vi "Profile_Write.vi"(8 "error in":errorcluster, 10 "Configuration Cluster":T1={"General"={"Config.ini"=path "", "Default Logging Path"=path ""}, "Hardware"={"LCR VISA COM"="", "Measure Rate (1/s)"=0, "Reset on Load?"=FALSE, "Measure Profile"=path "", "Global T VAR"="", "Global B VAR"=""}, "HM8118 Current Profile"={"Bias Profile"={" Bias Source (OFF)"=0, " Bias Type (Voltage)"=0, "Bias Level (0)"=0.0}, "Measurement Profile"={"Operation Mode (0: Auto)"=0, "Circuit Type (2: Auto)"=2, "Manual Range (1:Range 1 and 25 Ohms)"=1, "Auto Range (T: Enable)"=TRUE}, "Signal Profile"={"Frequency (1kHz)"=1000.0, "Measuring Voltage (1V)"=1.0}, "Integration Profile"={"Averaging (0: Off)"=0, "Averaging Number (2)"=2, "Time (100ms)"=100, "Rate (0: Fast)"=0}, "Trigger Profile"={"Trigger Mode (0: Continuous)"=0}}, "HM8118 New Profile"={"Bias Profile"={" Bias Source (OFF)"=0, " Bias Type (Voltage)"=0, "Bias Level (0)"=0.0}, "Measurement Profile"={"Operation Mode (0: Auto)"=0, "Circuit Type (2: Auto)"=2, "Manual Range (1:Range 1 and 25 Ohms)"=1, "Auto Range (T: Enable)"=TRUE}, "Signal Profile"={"Frequency (1kHz)"=1000.0, "Measuring Voltage (1V)"=1.0}, "Integration Profile"={"Averaging (0: Off)"=0, "Averaging Number (2)"=2, "Time (100ms)"=100, "Rate (0: Fast)"=0}, "Trigger Profile"={"Trigger Mode (0: Continuous)"=0}}, "Operation"={"Operation Mode"=enum."Idle-Off", "Status"="", "NewLog?"=FALSE}} {"HM8118 New Profile"."Trigger Profile"."Trigger Mode (0: Continuous)" items=["Continuous", "Manual", "External"]; "HM8118 New Profile"."Integration Profile"."Rate (0: Fast)" items=["Fast", "Medium", "Slow"]; "HM8118 New Profile"."Integration Profile"."Time (100ms)" min=1 max=999; "HM8118 New Profile"."Integration Profile"."Averaging Number (2)" min=2 max=99; "HM8118 New Profile"."Integration Profile"."Averaging (0: Off)" items=["Off", "Normal", "Averaging"]; "HM8118 New Profile"."Signal Profile"."Measuring Voltage (1V)" min=0.05 max=1.5 step=0.01; "HM8118 New Profile"."Signal Profile"."Frequency (1kHz)" min=20.0 max=200000.0; "HM8118 New Profile"."Measurement Profile"."Manual Range (1:Range 1 and 25 Ohms)" items=["Range 1 and 25 Ohms"=1, "Range 2 and 25 Ohms"=2, "Range 3 and 400 Ohms"=3, "Range 4 and 6.4 kOhms"=4, "Range 5 and 100kOhms"=5, "Range 6 and 100kOhms"=6]; "HM8118 New Profile"."Measurement Profile"."Circuit Type (2: Auto)" items=["Series", "Parallel", "Auto"]; "HM8118 New Profile"."Measurement Profile"."Operation Mode (0: Auto)" items=["Auto", "L+Q", "L+R", "C+D", "C+R", "R+Q", "Z+Theta", "Y+Theta", "R+X", "G+B", "N+Theta", "M"]; "HM8118 New Profile"."Bias Profile"."Bias Type (Voltage)" items=["Voltage", "Current"]; "HM8118 New Profile"."Bias Profile"."Bias Source (OFF)" items=["Off", "Internal", "External"]; "HM8118 Current Profile"."Trigger Profile"."Trigger Mode (0: Continuous)" items=["Continuous", "Manual", "External"]; "HM8118 Current Profile"."Integration Profile"."Rate (0: Fast)" items=["Fast", "Medium", "Slow"]; "HM8118 Current Profile"."Integration Profile"."Time (100ms)" min=1 max=999; "HM8118 Current Profile"."Integration Profile"."Averaging Number (2)" min=2 max=99; "HM8118 Current Profile"."Integration Profile"."Averaging (0: Off)" items=["Off", "Normal", "Averaging"]; "HM8118 Current Profile"."Signal Profile"."Measuring Voltage (1V)" min=0.05 max=1.5 step=0.01; "HM8118 Current Profile"."Signal Profile"."Frequency (1kHz)" min=20.0 max=200000.0; "HM8118 Current Profile"."Measurement Profile"."Manual Range (1:Range 1 and 25 Ohms)" items=["Range 1 and 25 Ohms"=1, "Range 2 and 25 Ohms"=2, "Range 3 and 400 Ohms"=3, "Range 4 and 6.4 kOhms"=4, "Range 5 and 100kOhms"=5, "Range 6 and 100kOhms"=6]; "HM8118 Current Profile"."Measurement Profile"."Circuit Type (2: Auto)" items=["Series", "Parallel", "Auto"]; "HM8118 Current Profile"."Measurement Profile"."Operation Mode (0: Auto)" items=["Auto", "L+Q", "L+R", "C+D", "C+R", "R+Q", "Z+Theta", "Y+Theta", "R+X", "G+B", "N+Theta", "M"]; "HM8118 Current Profile"."Bias Profile"."Bias Type (Voltage)" items=["Voltage", "Current"]; "HM8118 Current Profile"."Bias Profile"."Bias Source (OFF)" items=["Off", "Internal", "External"]}) -> (0 "error out":errorcluster, 2 "Configuration Cluster Out":T1={"General"={"Config.ini"=path "", "Default Logging Path"=path ""}, "Hardware"={"LCR VISA COM"="", "Measure Rate (1/s)"=0, "Reset on Load?"=FALSE, "Measure Profile"=path "", "Global T VAR"="", "Global B VAR"=""}, "HM8118 Current Profile"={"Bias Profile"={" Bias Source (OFF)"=0, " Bias Type (Voltage)"=0, "Bias Level (0)"=0.0}, "Measurement Profile"={"Operation Mode (0: Auto)"=0, "Circuit Type (2: Auto)"=2, "Manual Range (1:Range 1 and 25 Ohms)"=1, "Auto Range (T: Enable)"=TRUE}, "Signal Profile"={"Frequency (1kHz)"=1000.0, "Measuring Voltage (1V)"=1.0}, "Integration Profile"={"Averaging (0: Off)"=0, "Averaging Number (2)"=2, "Time (100ms)"=100, "Rate (0: Fast)"=0}, "Trigger Profile"={"Trigger Mode (0: Continuous)"=0}}, "HM8118 New Profile"={"Bias Profile"={" Bias Source (OFF)"=0, " Bias Type (Voltage)"=0, "Bias Level (0)"=0.0}, "Measurement Profile"={"Operation Mode (0: Auto)"=0, "Circuit Type (2: Auto)"=2, "Manual Range (1:Range 1 and 25 Ohms)"=1, "Auto Range (T: Enable)"=TRUE}, "Signal Profile"={"Frequency (1kHz)"=1000.0, "Measuring Voltage (1V)"=1.0}, "Integration Profile"={"Averaging (0: Off)"=0, "Averaging Number (2)"=2, "Time (100ms)"=100, "Rate (0: Fast)"=0}, "Trigger Profile"={"Trigger Mode (0: Continuous)"=0}}, "Operation"={"Operation Mode"=enum."Idle-Off", "Status"="", "NewLog?"=FALSE}} {"HM8118 New Profile"."Trigger Profile"."Trigger Mode (0: Continuous)" items=["Continuous", "Manual", "External"]; "HM8118 New Profile"."Integration Profile"."Rate (0: Fast)" items=["Fast", "Medium", "Slow"]; "HM8118 New Profile"."Integration Profile"."Time (100ms)" min=1 max=999; "HM8118 New Profile"."Integration Profile"."Averaging Number (2)" min=2 max=99; "HM8118 New Profile"."Integration Profile"."Averaging (0: Off)" items=["Off", "Normal", "Averaging"]; "HM8118 New Profile"."Signal Profile"."Measuring Voltage (1V)" min=0.05 max=1.5 step=0.01; "HM8118 New Profile"."Signal Profile"."Frequency (1kHz)" min=20.0 max=200000.0; "HM8118 New Profile"."Measurement Profile"."Manual Range (1:Range 1 and 25 Ohms)" items=["Range 1 and 25 Ohms"=1, "Range 2 and 25 Ohms"=2, "Range 3 and 400 Ohms"=3, "Range 4 and 6.4 kOhms"=4, "Range 5 and 100kOhms"=5, "Range 6 and 100kOhms"=6]; "HM8118 New Profile"."Measurement Profile"."Circuit Type (2: Auto)" items=["Series", "Parallel", "Auto"]; "HM8118 New Profile"."Measurement Profile"."Operation Mode (0: Auto)" items=["Auto", "L+Q", "L+R", "C+D", "C+R", "R+Q", "Z+Theta", "Y+Theta", "R+X", "G+B", "N+Theta", "M"]; "HM8118 New Profile"."Bias Profile"."Bias Type (Voltage)" items=["Voltage", "Current"]; "HM8118 New Profile"."Bias Profile"."Bias Source (OFF)" items=["Off", "Internal", "External"]; "HM8118 Current Profile"."Trigger Profile"."Trigger Mode (0: Continuous)" items=["Continuous", "Manual", "External"]; "HM8118 Current Profile"."Integration Profile"."Rate (0: Fast)" items=["Fast", "Medium", "Slow"]; "HM8118 Current Profile"."Integration Profile"."Time (100ms)" min=1 max=999; "HM8118 Current Profile"."Integration Profile"."Averaging Number (2)" min=2 max=99; "HM8118 Current Profile"."Integration Profile"."Averaging (0: Off)" items=["Off", "Normal", "Averaging"]; "HM8118 Current Profile"."Signal Profile"."Measuring Voltage (1V)" min=0.05 max=1.5 step=0.01; "HM8118 Current Profile"."Signal Profile"."Frequency (1kHz)" min=20.0 max=200000.0; "HM8118 Current Profile"."Measurement Profile"."Manual Range (1:Range 1 and 25 Ohms)" items=["Range 1 and 25 Ohms"=1, "Range 2 and 25 Ohms"=2, "Range 3 and 400 Ohms"=3, "Range 4 and 6.4 kOhms"=4, "Range 5 and 100kOhms"=5, "Range 6 and 100kOhms"=6]; "HM8118 Current Profile"."Measurement Profile"."Circuit Type (2: Auto)" items=["Series", "Parallel", "Auto"]; "HM8118 Current Profile"."Measurement Profile"."Operation Mode (0: Auto)" items=["Auto", "L+Q", "L+R", "C+D", "C+R", "R+Q", "Z+Theta", "Y+Theta", "R+X", "G+B", "N+Theta", "M"]; "HM8118 Current Profile"."Bias Profile"."Bias Type (Voltage)" items=["Voltage", "Current"]; "HM8118 Current Profile"."Bias Profile"."Bias Source (OFF)" items=["Off", "Internal", "External"]})   [LabVIEW 2021]
uses:
  Config_Cluster.ctl
  Mode_Enum.ctl
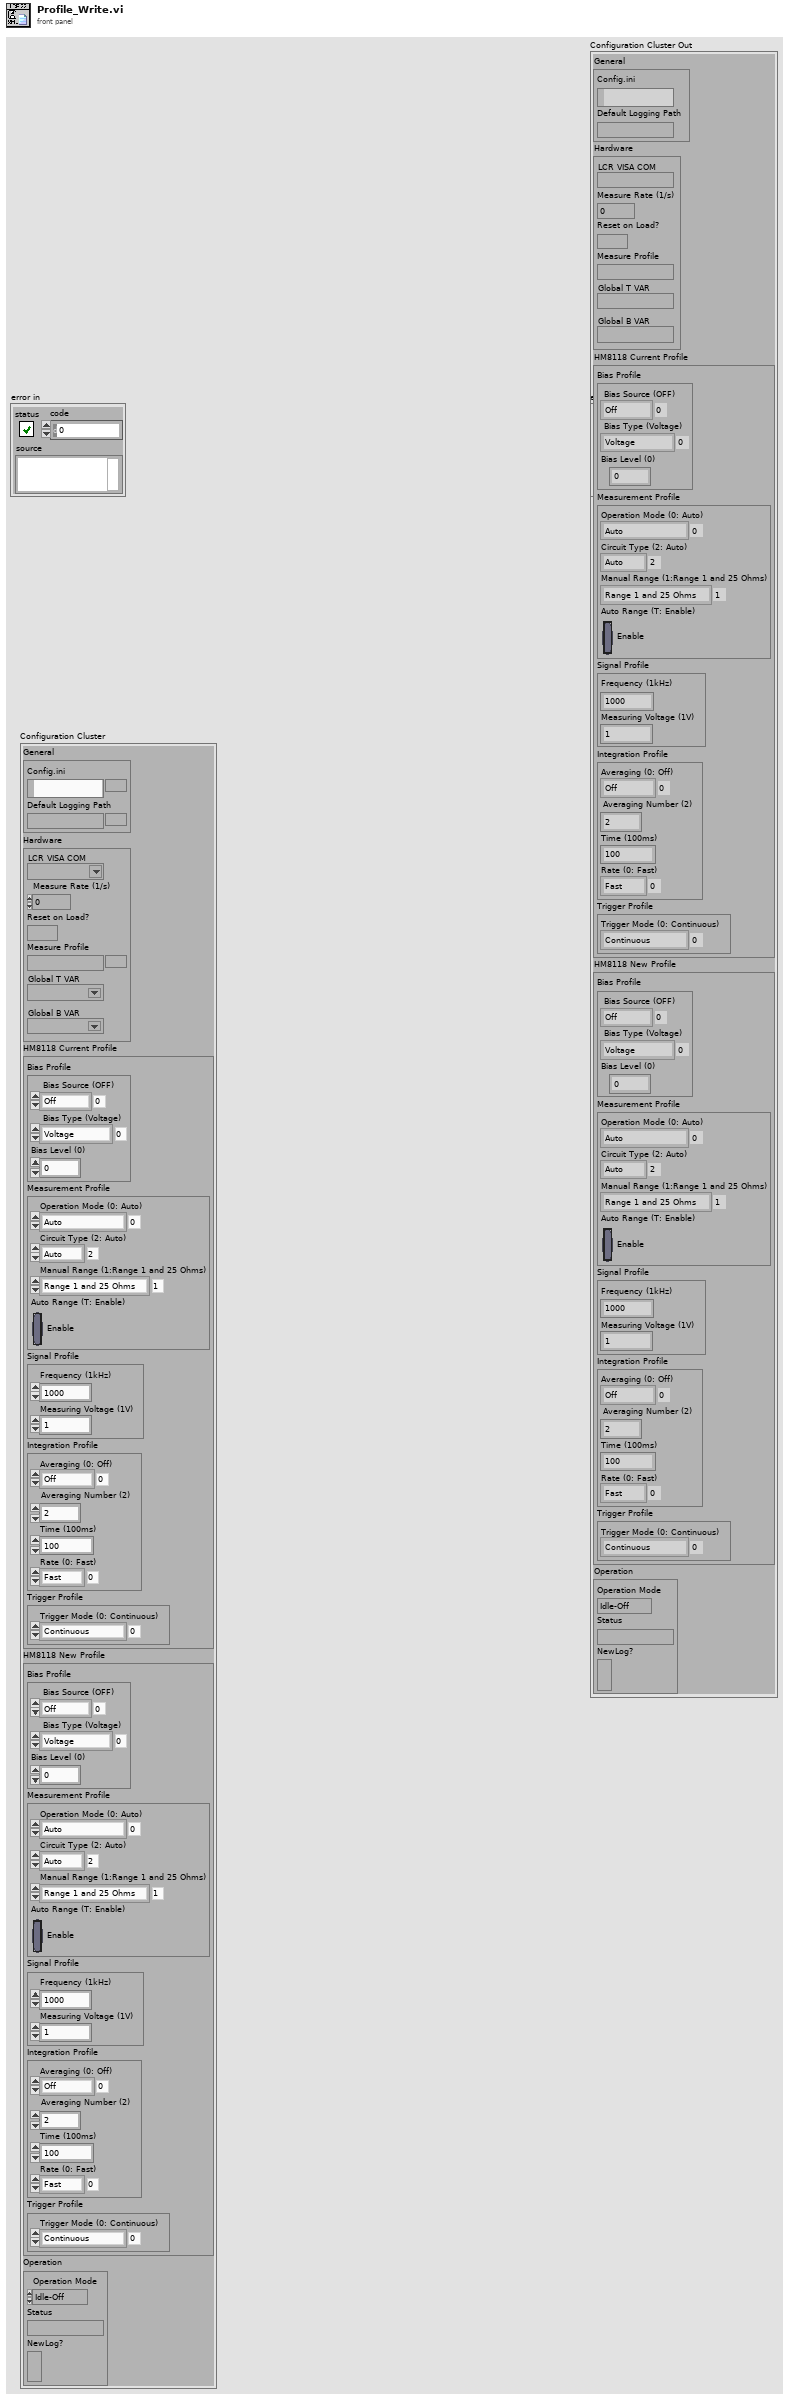
[diagram p1: front panel]
types:
  T1 = typedef "Config_Cluster.ctl" = cluster{"General":cluster{"Config.ini":path, "Default Logging Path":path}, "Hardware":cluster{"LCR VISA COM":refnum<visa-resource-name>, "Measure Rate (1/s)":i32, "Reset on Load?":bool, "Measure Profile":path, "Global T VAR":refnum<k21>, "Global B VAR":refnum<k21>}, "HM8118 Current Profile":cluster{"Bias Profile":cluster{" Bias Source (OFF)":u8, " Bias Type (Voltage)":u8, "Bias Level (0)":dbl}, "Measurement Profile":cluster{"Operation Mode (0: Auto)":u16, "Circuit Type (2: Auto)":u16, "Manual Range (1:Range 1 and 25 Ohms)":u8, "Auto Range (T: Enable)":bool}, "Signal Profile":cluster{"Frequency (1kHz)":dbl, "Measuring Voltage (1V)":dbl}, "Integration Profile":cluster{"Averaging (0: Off)":u16, "Averaging Number (2)":i32, "Time (100ms)":i32, "Rate (0: Fast)":u16}, "Trigger Profile":cluster{"Trigger Mode (0: Continuous)":u16}}, "HM8118 New Profile":cluster{"Bias Profile":cluster{" Bias Source (OFF)":u8, " Bias Type (Voltage)":u8, "Bias Level (0)":dbl}, "Measurement Profile":cluster{"Operation Mode (0: Auto)":u16, "Circuit Type (2: Auto)":u16, "Manual Range (1:Range 1 and 25 Ohms)":u8, "Auto Range (T: Enable)":bool}, "Signal Profile":cluster{"Frequency (1kHz)":dbl, "Measuring Voltage (1V)":dbl}, "Integration Profile":cluster{"Averaging (0: Off)":u16, "Averaging Number (2)":i32, "Time (100ms)":i32, "Rate (0: Fast)":u16}, "Trigger Profile":cluster{"Trigger Mode (0: Continuous)":u16}}, "Operation":cluster{"Operation Mode":T2, "Status":string, "NewLog?":bool}}
  T2 = typedef "Mode_Enum.ctl" = enum16{"Logging", "Idle-Off", "Idle"}
  T3 = enum16{"open", "replace", "create", "open or create", "replace or create", "replace or create with confirmation"}
  T4 = cluster{"Bias Profile":cluster{" Bias Source (OFF)":u8, " Bias Type (Voltage)":u8, "Bias Level (0)":dbl}, "Measurement Profile":cluster{"Operation Mode (0: Auto)":u16, "Circuit Type (2: Auto)":u16, "Manual Range (1:Range 1 and 25 Ohms)":u8, "Auto Range (T: Enable)":bool}, "Signal Profile":cluster{"Frequency (1kHz)":dbl, "Measuring Voltage (1V)":dbl}, "Integration Profile":cluster{"Averaging (0: Off)":u16, "Averaging Number (2)":i32, "Time (100ms)":i32, "Rate (0: Fast)":u16}, "Trigger Profile":cluster{"Trigger Mode (0: Continuous)":u16}}
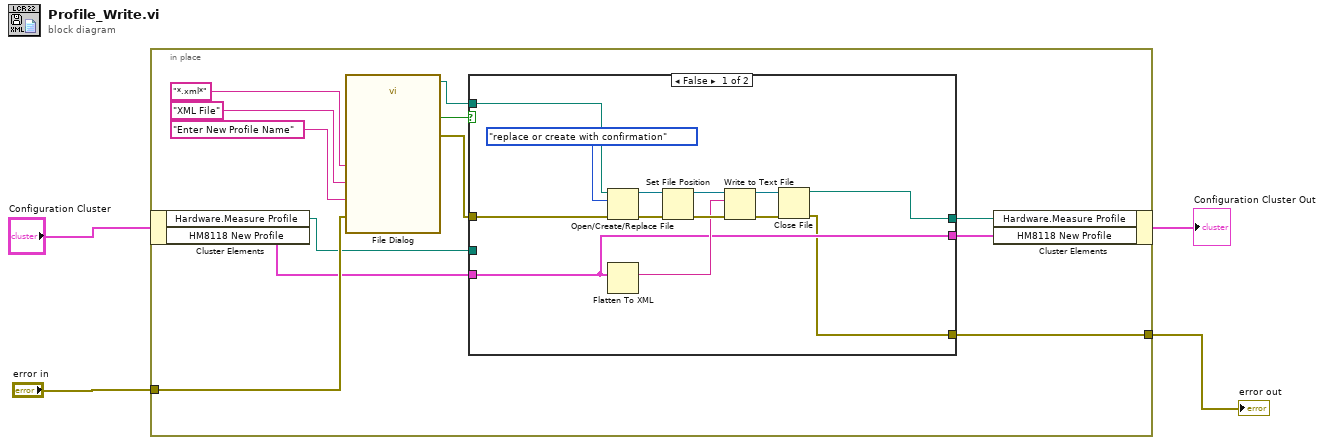
[diagram p0: block diagram]
diagram:
  n1 = in-place {
    in-place-border: "error in" -> [w11]
    in-place-border: [w5] -> w2
    n2 = in-place-cluster #1("Configuration Cluster") -> ("Hardware.Measure Profile"=w6:path, "HM8118 New Profile"=w9:T4)
    n3 = call "File Dialog"("prompt"="Enter New Profile Name", "error in"=w11, "pattern (all files)"="*.xml*", "pattern label"="XML File") -> ("selected path"=w12:path, "cancelled"=w13:bool, "error out"=w10:errorcluster)  [unwired: 8 in, 1 out]
    n4 = case shown="False" w13 {
      tunnel: w12 -> [w29 _]
      tunnel: w10 -> [w27 w30]
      tunnel: w9 -> [w18 w31]
      tunnel: [w19 w32] -> w8
      tunnel: [w18 w31] -> w7
      tunnel: w6 -> [_ w32]
      tunnel: [w17 w30] -> w5
      frame False {
        n5 = Open/Create/Replace File(file path (use dialog)=w29, error in=w27, operation (0:open)=T3."replace or create with confirmation") -> (refnum out=w26:refnum<file>, error out=w25:errorcluster)  [unwired: 3 in, 1 out]
        n6 = Flatten To XML(6:w18) -> (2:w22:string)
        n7 = Set File Position(refnum=w26, error in=w25) -> (refnum out=w24:refnum<file>, error out=w23:errorcluster)  [unwired: 2 in]
        n8 = Write to Text File(file (use dialog)=w24, text=w22, error in=w23) -> (refnum out=w20:refnum<file>, error out=w21:errorcluster)  [unwired: 1 in, 1 out]
        n9 = Close File(refnum=w20, error in=w21) -> (path=w19:path, error out=w17:errorcluster)
      }
      frame True {
      }
    }
    n10 = in-place-cluster #1("Hardware.Measure Profile"=w8, "HM8118 New Profile"=w7) -> (→"Configuration Cluster Out":T1)
  }
  "error out" <- w2
